vi "fetchReport.vi"(8 "Error In":errorcluster, 11 "UI Elements Cluster":T1) -> (0 "Error Out":errorcluster, 3 "Report":string[][](array[string]))   [LabVIEW 2018]
uses:
  UI Module/src/controls/mainAppElementsCluster.ctl
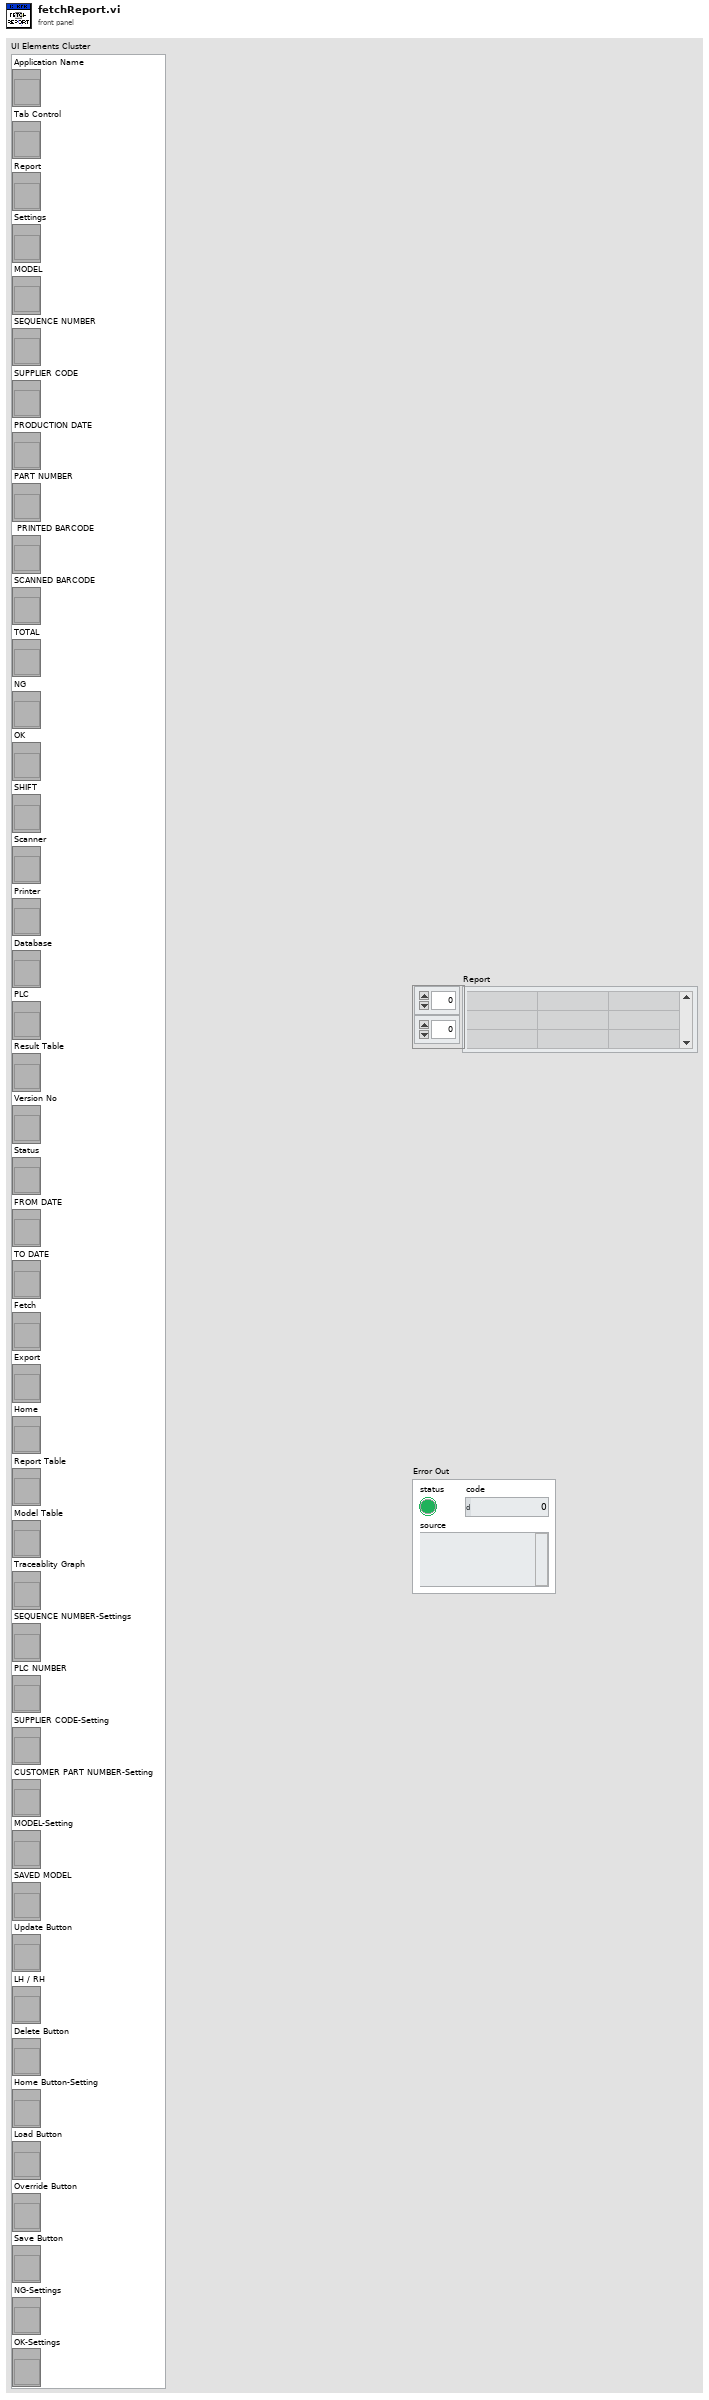
[diagram p1: front panel]
types:
  T1 = typedef "mainAppElementsCluster.ctl" = cluster{"Application Name":refnum<vi>, "Tab Control":refnum<vi>, "Status":refnum<vi>, "Version No":refnum<vi>, "Result Table":refnum<vi>, "PLC":refnum<vi>, "Database":refnum<vi>, "Printer":refnum<vi>, "Scanner":refnum<vi>, "SHIFT":refnum<vi>, "OK":refnum<vi>, "NG":refnum<vi>, "TOTAL":refnum<vi>, "SCANNED BARCODE":refnum<vi>, " PRINTED BARCODE":refnum<vi>, "PART NUMBER":refnum<vi>, "PRODUCTION DATE":refnum<vi>, "SUPPLIER CODE":refnum<vi>, "SEQUENCE NUMBER":refnum<vi>, "MODEL":refnum<vi>, "Settings":refnum<vi>, "Report":refnum<vi>, "Report Table":refnum<vi>, "Home":refnum<vi>, "Export":refnum<vi>, "Fetch":refnum<vi>, "TO DATE":refnum<vi>, "FROM DATE":refnum<vi>, "Model Table":refnum<vi>, "Traceablity Graph":refnum<vi>, "Override Button":refnum<vi>, "Load Button":refnum<vi>, "Home Button-Setting":refnum<vi>, "Delete Button":refnum<vi>, "Update Button":refnum<vi>, "Save Button":refnum<vi>, "SEQUENCE NUMBER-Settings":refnum<vi>, "PLC NUMBER":refnum<vi>, "LH / RH":refnum<vi>, "SUPPLIER CODE-Setting":refnum<vi>, "CUSTOMER PART NUMBER-Setting":refnum<vi>, "MODEL-Setting":refnum<vi>, "SAVED MODEL":refnum<vi>, "NG-Settings":refnum<vi>, "OK-Settings":refnum<vi>}
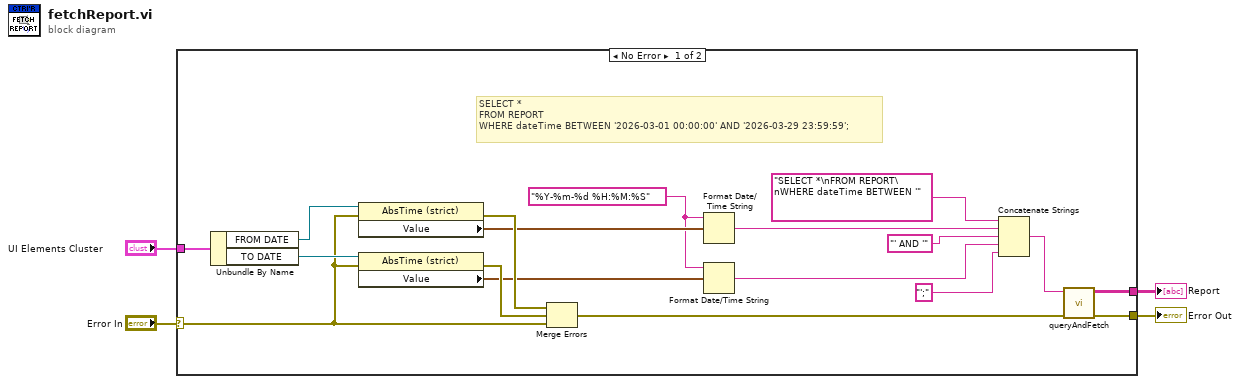
[diagram p0: block diagram]
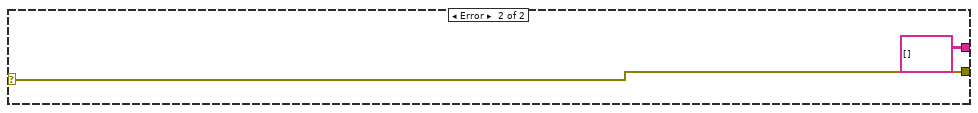
[diagram p2: hidden frame]
diagram:
  n1 = case shown="No Error" "Error In" {
    selector: "Error In" -> [w18 w24]
    tunnel: [w21 w24] -> w4
    tunnel: "UI Elements Cluster" -> [w22 _]
    tunnel: [w5 string[][] [] ("Result Table")] -> w1
    frame No Error {
      w12 = "%Y-%m-%d %H:%M:%S" ("time format string (%c)")
      # "SELECT *\nFROM REPORT\nWHERE dateTime BETWEEN '2026-03-01 00:00:00' AND '2026-03-29 23:59:59';"
      n2 = Unbundle By Name(w22) -> ("FROM DATE"=w20:refnum<vi>, "TO DATE"=w19:refnum<vi>)
      n3 = property class="AbsTime (strict)"(reference=w20, error in=w18) -> (error out=w15:errorcluster, "Value"=w14:timestamp)  [unwired: 1 out]
      n4 = property class="AbsTime (strict)"(reference=w19, error in=w18) -> (error out=w16:errorcluster, "Value"=w13:timestamp)  [unwired: 1 out]
      n5 = Merge Errors(w15, w16, w18) -> (w17:errorcluster)
      n6 = Format Date/Time String(time format string (%c)=w12, seconds (now)=w14) -> (date/time string=w9:string)  [unwired: 1 in]
      n7 = Format Date/Time String(time format string (%c)=w12, seconds (now)=w13) -> (date/time string=w7:string)  [unwired: 1 in]
      n8 = Concatenate Strings("SELECT *\nFROM REPORT\nWHERE dateTime BETWEEN '", w9, "' AND '", w7, "';") -> (w10:string)
      n9 = call "queryAndFetch.vi"("Error In"=w17, "Query"=w10) -> ("Error Out"=w21:errorcluster, "Result Table"=w5:string[][])  [unwired: 8 in]
    }
    frame Error {
    }
  }
  "Error Out" <- w4
  "Report" <- w1
